vi "Queue Last Ack.vi"(10 "Queue Actor":refnum<class "Queue Actor.lvclass">, 11 "jettl Queue Actor in":refnum<class "jettl Queue Actor.lvclass">) -> (3 "jettl Queue Actor out":refnum<class "jettl Queue Actor.lvclass">)   [LabVIEW 2021, in "jettl.lvlib" / "jettl Queue Actor.lvlib" / "jettl Queue Actor.lvclass"]
uses:
  jettl Queue Actor.lvclass
  Actor/Queue Actor/Queue Actor.lvclass
  jettl Queue Actor.lvclass/jettl Queue Actor.ctl
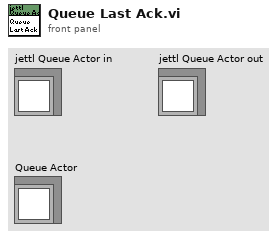
[diagram p1: front panel]
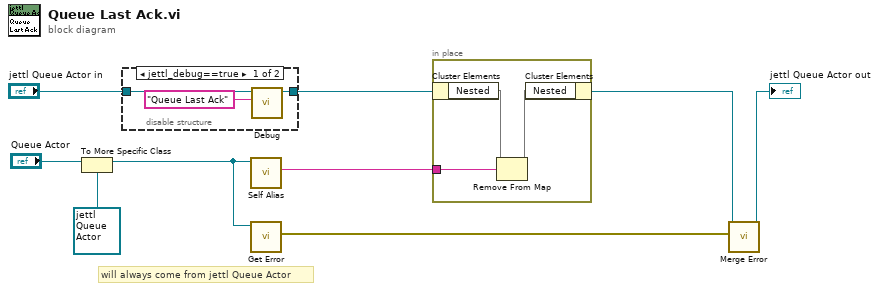
[diagram p0: block diagram]
diagram:
  # "will always come from jettl Queue Actor"
  n1 = To More Specific Class(target class=refnum<class "jettl Queue Actor.lvclass"> refnum ("jettl.lvlib:jettl Queue Actor.lvlib:jettl Queue Actor.lvclass"), reference="Queue Actor") -> (specific class reference=w4:refnum<class "jettl Queue Actor.lvclass">)  [unwired: 1 in, 1 out]
  n2 = disable-structure shown="jettl_debug==true" {
    disable-tunnel: "jettl Queue Actor in" -> [w12 w13]
    disable-tunnel: [w11 w13] -> w2
    frame condition #0 (active) {
      n3 = call "Debug.vi"("Method"="Queue Last Ack", "jettl Queue Actor in"=w12) -> ("jettl Queue Actor out"=w11:refnum<class "jettl Queue Actor.lvclass">)  [unwired: 9 in]
    }
    frame condition #1 {
    }
  }
  n4 = call-dynamic "Self Alias.vi"("jettl Queue Actor in"=w4) -> ("Self Alias"=w5:string)  [unwired: 10 in]
  n5 = call-dynamic "Get Error.vi"("jettl Queue Actor in"=w4) -> ("Error"=w3:errorcluster)  [unwired: 10 in]
  n6 = in-place {
    in-place-border: w5 -> [w14]
    n7 = in-place-cluster #1(w2) -> ("Nested"=w15:map{string, refnum<data-value>})
    n8 = Remove From Map(10:w14, 11:w15) -> (3:w16:map{string, refnum<data-value>})  [unwired: 2 out]
    n9 = in-place-cluster #1("Nested"=w16) -> (w1:refnum<class "jettl Queue Actor.lvclass">)
  }
  n10 = call-dynamic "Merge Error.vi"("Error"=w3, "jettl Queue Actor in"=w1) -> ("jettl Queue Actor out"=→"jettl Queue Actor out":refnum<class "jettl Queue Actor.lvclass">)  [unwired: 9 in]
